vi "testWrongDataSet.vi"() -> ()   [LabVIEW 2017, in "TheoryTest.lvlib"]
uses:
  TheoryTest.lvlib
  Theory/Theory.lvclass
  Support/Support.lvlib
  Assertion/Assertion.lvlib
  ControlData.ctl
panel:
  out "error out":errorcluster
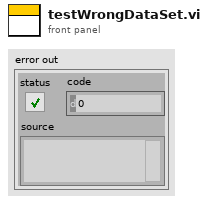
[diagram p1: front panel]
types:
  T1 = typedef "ControlData.ctl" = cluster{"Name":string, "Data":variant}
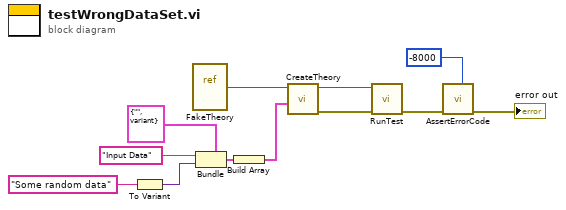
[diagram p0: block diagram]
diagram:
  n1 = To Variant(anything="Some random data" ("key")) -> (Variant=w5:variant)
  n2 = vi-ref "FakeTheory.vi"() -> (w3:refnum<vi>)
  n3 = Bundle(cluster=T1 {"Name"="", "Data"=variant} ("Control Data"), "Name"="Input Data" ("key"), "Data"=w5) -> (w6:T1)
  n4 = Build Array(w6) -> (w1:T1[])
  n5 = call "CreateTheory.vi"("Control Data"=w1, "VI Refnum"=w3) -> ("error out"=w11:errorcluster, "Theory"=w12:refnum<class "Theory.lvclass">)  [unwired: 8 in]
  n6 = call-dynamic "RunTest.vi"("error in (no error)"=w11, "Theory in"=w12) -> ("error out"=w10:errorcluster)  [unwired: 8 in, 1 out]
  n7 = call "AssertErrorCode.vi"("Expected"=-8000, "error in (no error)"=w10) -> ("error out"=→"error out":errorcluster)  [unwired: 9 in]
